vi "Get measuring exp.vi"(8 "error in (no error)":errorcluster, 11 "Control-Client in":refnum<class "Control-Client.lvclass">) -> (0 "error out":errorcluster, 2 "Measured experiment":refnum<class "Experiment.lvclass">, 3 "Control-Client out":refnum<class "Control-Client.lvclass">)   [LabVIEW 2018, in "Control-Client.lvclass"]
uses:
  Control-Client.lvclass
  Experiments/Experiment.lvclass
  Control-Client.lvclass/Control-Client.ctl
  methods/Read Group #.vi
  Experiments/Experiments_group.lvclass
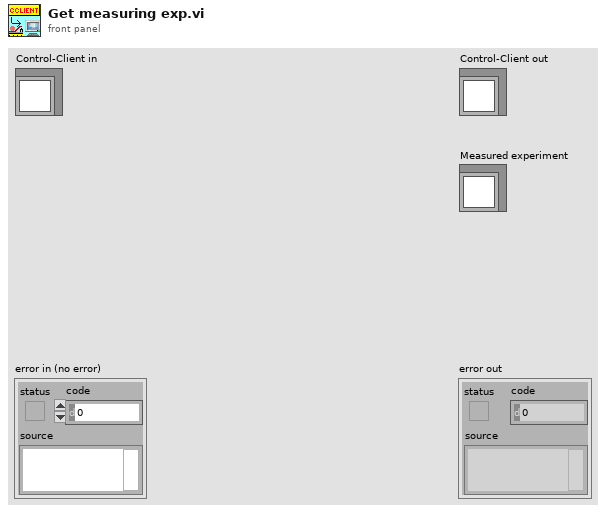
[diagram p1: front panel]
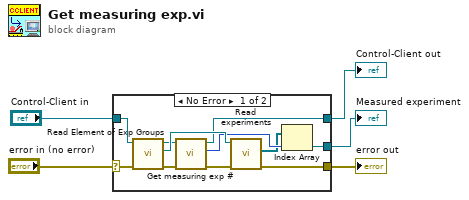
[diagram p0: block diagram]
diagram:
  n1 = case shown="No Error" "error in (no error)" {
    selector: "error in (no error)" -> [w16 w18]
    tunnel: [w6 w18] -> w4
    tunnel: [w9 w17] -> w2
    tunnel: "Control-Client in" -> [w11 w17]
    tunnel: [w12 _] -> w1
    frame No Error {
      n2 = call "Read Element of Exp Groups.vi"("error in (no error)"=w16, "Control-Client in"=w11) -> ("error out"=w8:errorcluster, "Experiments_group.lvclass"=w15:refnum<class "Experiments_group.lvclass">, "Control-Client out"=w10:refnum<class "Control-Client.lvclass">)  [unwired: 7 in]
      n3 = call "Get measuring exp #.vi"("error in (no error)"=w8, "Control-Client in"=w10) -> ("error out"=w7:errorcluster, "Exp measure #"=w14:i32, "Control-Client out"=w9:refnum<class "Control-Client.lvclass">)  [unwired: 7 in]
      n4 = call "Read experiments.vi"("error in (no error)"=w7, "Experiments_group.lvclass in"=w15) -> ("error out"=w6:errorcluster, "Experiments"=w13:refnum<class "Experiment.lvclass">[])  [unwired: 6 in, 1 out]
      n5 = Index Array(array=w13, index=w14) -> (element=w12:refnum<class "Experiment.lvclass">)
    }
    frame Error {
    }
  }
  "error out" <- w4
  "Control-Client out" <- w2
  "Measured experiment" <- w1
